vi "Autonomous.vi"   [LabVIEW 2015]
doc: "This VI starts when autonomous period begins, and will automatically be terminated when it ends. You can carry out timed or sensor driven operations directly to I/O or to subsystems without needing to return to the caller."
uses:
  <vilib>/Rock Robotics/WPI/CAN/TalonSRX/WPI_CANTalonSRX_Params.ctl
  <vilib>/Rock Robotics/Network Tables/NT Read Number.vi
  <vilib>/Rock Robotics/Network Tables/NT Read Boolean.vi
  Drive/Implementation/Drive Published Globals.vi
  Intake/Implementation/Intake Published Globals.vi
  Turret/Implementation/Turret Published Globals.vi
types:
  T1 = typedef "WPI_MotorControlDeviceRef.ctl" = cluster{"DeviceStatus":errorcluster, "Type":T2, "PWM":cluster{"PWM Channel":T3, "DeadBand":T4}, "CAN":cluster{"Device Number":u8, "Control Mode":T5, "Semaphore":T6, "Max Vout":dbl, "TalonSRX Control Mode":T7}, "Invert":bool}
  T2 = typedef "WPI_MotorControlType.ctl" = enum16{"PWM", "CAN", "CANTalonSRX"}
  T3 = typedef "FPGA_DIOPWMChannel.ctl" = enum8{"PWM 0", "PWM 1", "PWM 2", "PWM 3", "PWM 4", "PWM 5", "PWM 6", "PWM 7", "PWM 8", "PWM 9", "PWM MXP 0", "PWM MXP 1", "PWM MXP 2", "PWM MXP 3", "PWM MXP 4", "PWM MXP 5", "PWM MXP 6", "PWM MXP 7", "PWM MXP 8", "PWM MXP 9", "Invalid"}
  T4 = typedef "WPI_PWMDeadband.ctl" = cluster{"Name":string, "maxPositivePwm":i32, "minPositivePwm":i32, "centerPwm":i32, "maxNegativePwm":i32, "minNegativePwm":i32, "angularRange":u16}
  T5 = typedef "WPI_CANJaguar_ControlMode.ctl" = enum8{"Percent VBus", "Current", "Speed", "Position", "Voltage"}
  T6 = typedef "Semaphore RefNum" = refnum<k1>
  T7 = typedef "WPI_CANTalonSRX_APIControlMode.ctl" = enum8{"Percent VBus", "Speed", "Position", "Slave", "Unchanged / Invalid", "Voltage Compensation", "Current", "Motion Profile"}
  T8 = typedef "WPI_CANTalonSRX_Params.ctl" = u8
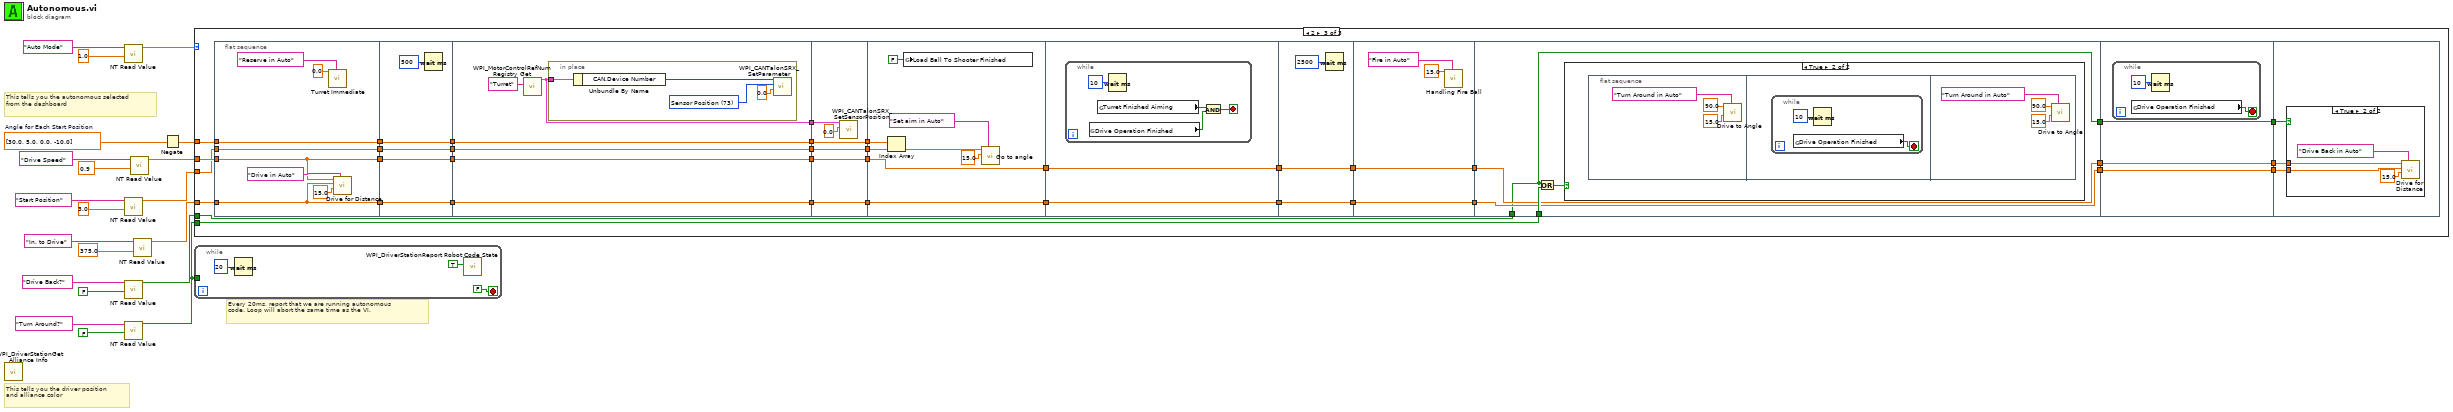
[diagram p0: block diagram]
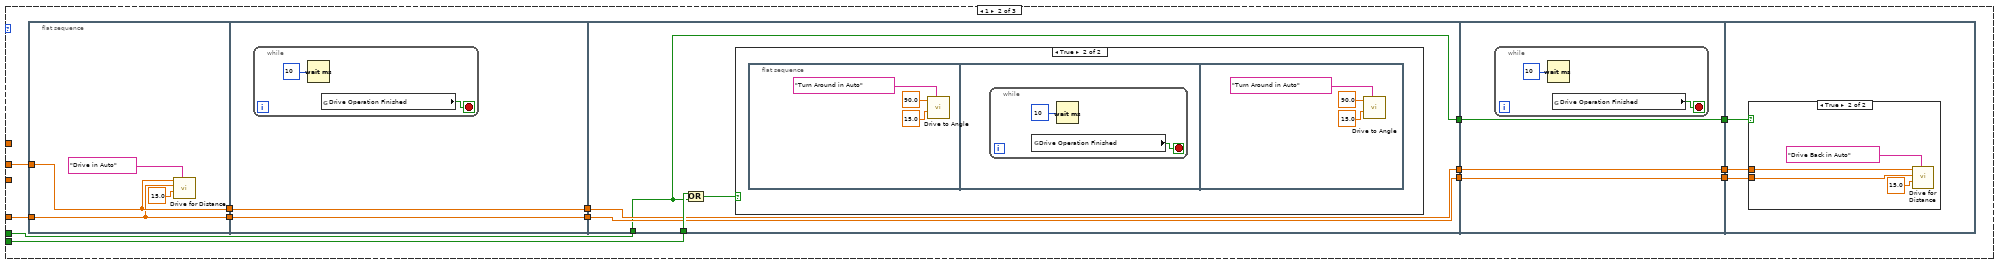
[diagram p3: hidden frame]
diagram:
  w13 = dbl[] [30.0, 5.0, 0.0, -10.0]  # Angle for Each Start Position
  # "This tells you the autonomous selected\nfrom the dashboard"
  # "Every 20ms, report that we are running autonomous\ncode. Loop will abort the same time as the VI."
  # "This tells you the driver position\nand alliance color"
  n1 = call <vilib>:"WPI_DriverStationGet Alliance Info.vi"() -> ()  [unwired: 12 out]
  n2 = call-poly <vilib>:"NT Read Value.vi"("Default Value"=1.0, "Name"="Auto Mode") -> ("Numeric"=w19:dbl)  [unwired: 8 in, 1 out]
  n3 = call-poly <vilib>:"NT Read Value.vi"("Default Value"=3.0, "Name"="Start Position") -> ("Numeric"=w12:dbl)  [unwired: 8 in, 1 out]
  n4 = call-poly <vilib>:"NT Read Value.vi"("Default Value"=FALSE, "Name"="Drive Back?") -> ("Boolean"=w3:bool)  [unwired: 8 in, 1 out]
  n5 = call-poly <vilib>:"NT Read Value.vi"("Default Value"=FALSE, "Name"="Turn Around?") -> ("Boolean"=w1:bool)  [unwired: 8 in, 1 out]
  n6 = call-poly <vilib>:"NT Read Value.vi"("Default Value"=0.9, "Name"="Drive Speed") -> ("Numeric"=w15:dbl)  [unwired: 8 in, 1 out]
  n7 = call-poly <vilib>:"NT Read Value.vi"("Default Value"=375.0, "Name"="In. to Drive") -> ("Numeric"=w17:dbl)  [unwired: 8 in, 1 out]
  n8 = Negate(x=w13) -> (-x=w2:dbl[])
  n9 = case shown="2" w19 {
    tunnel: w17 -> [_ w34 w103]
    tunnel: w15 -> [_ w33 w104]
    tunnel: w2 -> [_ _ w102]
    tunnel: w12 -> [_ _ w101]
    tunnel: w1 -> [_ w32 w99]
    tunnel: w3 -> [_ w31 w100]
    frame 0, Default {
    }
    frame 1 {
      n10 = flat-sequence {
        tunnel: w34 -> [w35]
        tunnel: w33 -> [w36]
        tunnel: [w36] -> w30
        tunnel: [w35] -> w28
        tunnel: w30 -> [w40]
        tunnel: [w40] -> w29
        tunnel: w28 -> [w39]
        tunnel: [w39] -> w27
        tunnel: w32 -> [w47]
        tunnel: w31 -> [w44]
        tunnel: w29 -> [w46]
        tunnel: [w46] -> w26
        tunnel: w27 -> [w45]
        tunnel: [w45] -> w24
        tunnel: [w44] -> w22
        tunnel: w26 -> [w58]
        tunnel: [w58] -> w25
        tunnel: w24 -> [w57]
        tunnel: [w57] -> w23
        tunnel: w22 -> [w56]
        tunnel: [w56] -> w21
        tunnel: w25 -> [w63]
        tunnel: w23 -> [w62]
        tunnel: w21 -> [w61]
        frame #0 {
          n11 = call "Drive for Distance.vi"("Description"="Drive in Auto", "Duration"=15.0, "Distance (in.)"=w35, "Speed (-1 to 1)"=w36) -> ()  [unwired: 7 in, 1 out]
        }
        frame #1 {
          n12 = while {
            stop <- w41 stop-if-true
            n13 = Wait (ms)(milliseconds to wait=10) -> ()  [unwired: 1 out]
            n14 = global read "Drive Published Globals.vi" "Drive Operation Finished"() -> (w41:bool)
          }
        }
        frame #2 {
          n15 = Or(x=w47, y=w44) -> (x .or. y?=w43:bool)
          n16 = case shown="True" w43 {
            frame False {
            }
            frame True {
              n17 = flat-sequence {
                frame #0 {
                  n18 = call "Drive to Angle.vi"("Description"="Turn Around in Auto", "Duration"=15.0, "Angle"=90.0) -> ()  [unwired: 8 in, 1 out]
                }
                frame #1 {
                  n19 = while {
                    stop <- w51 stop-if-true
                    n20 = global read "Drive Published Globals.vi" "Drive Operation Finished"() -> (w51:bool)
                    n21 = Wait (ms)(milliseconds to wait=10) -> ()  [unwired: 1 out]
                  }
                }
                frame #2 {
                  n22 = call "Drive to Angle.vi"("Description"="Turn Around in Auto", "Duration"=15.0, "Angle"=90.0) -> ()  [unwired: 8 in, 1 out]
                }
              }
            }
          }
        }
        frame #3 {
          n23 = while {
            stop <- w59 stop-if-true
            n24 = Wait (ms)(milliseconds to wait=10) -> ()  [unwired: 1 out]
            n25 = global read "Drive Published Globals.vi" "Drive Operation Finished"() -> (w59:bool)
          }
        }
        frame #4 {
          n26 = case shown="True" w61 {
            tunnel: w63 -> [_ w65]
            tunnel: w62 -> [_ w64]
            frame False {
            }
            frame True {
              n27 = call "Drive for Distance.vi"("Description"="Drive Back in Auto", "Duration"=15.0, "Distance (in.)"=w64, "Speed (-1 to 1)"=w65) -> ()  [unwired: 7 in, 1 out]
            }
          }
        }
      }
    }
    frame 2 {
      n28 = flat-sequence {
        tunnel: w101 -> [w111]
        tunnel: w102 -> [w112]
        tunnel: w103 -> [w108]
        tunnel: w104 -> [w107]
        tunnel: [w107] -> w84
        tunnel: [w108] -> w82
        tunnel: [w112] -> w80
        tunnel: [w111] -> w78
        tunnel: w84 -> [w117]
        tunnel: [w117] -> w83
        tunnel: w82 -> [w116]
        tunnel: [w116] -> w81
        tunnel: w80 -> [w115]
        tunnel: [w115] -> w79
        tunnel: w78 -> [w114]
        tunnel: [w114] -> w77
        tunnel: [w123] -> w76
        tunnel: [w122] -> w74
        tunnel: [w121] -> w72
        tunnel: [w120] -> w70
        tunnel: w83 -> [w123]
        tunnel: w81 -> [w122]
        tunnel: w79 -> [w121]
        tunnel: w77 -> [w120]
        tunnel: [w118] -> w68
        tunnel: w76 -> [w133]
        tunnel: [w133] -> w75
        tunnel: w74 -> [w132]
        tunnel: [w132] -> w73
        tunnel: w72 -> [w131]
        tunnel: [w131] -> w71
        tunnel: w70 -> [w130]
        tunnel: [w130] -> w69
        tunnel: w68 -> [w129]
        tunnel: w75 -> [w135]
        tunnel: w73 -> [w134]
        tunnel: w71 -> [w141]
        tunnel: w69 -> [w140]
        tunnel: [w135] -> w95
        tunnel: [w134] -> w91
        tunnel: [w143] -> w96
        tunnel: w95 -> [w143]
        tunnel: [w142] -> w92
        tunnel: w91 -> [w142]
        tunnel: [w149] -> w97
        tunnel: w96 -> [w149]
        tunnel: [w148] -> w93
        tunnel: w92 -> [w148]
        tunnel: [w152] -> w98
        tunnel: w97 -> [w152]
        tunnel: [w151] -> w94
        tunnel: w93 -> [w151]
        tunnel: w100 -> [w155]
        tunnel: w99 -> [w158]
        tunnel: w98 -> [w157]
        tunnel: w94 -> [w156]
        tunnel: [w155] -> w90
        tunnel: [w157] -> w89
        tunnel: [w156] -> w88
        tunnel: w90 -> [w170]
        tunnel: [w170] -> w87
        tunnel: w89 -> [w169]
        tunnel: [w169] -> w86
        tunnel: w88 -> [w168]
        tunnel: [w168] -> w85
        tunnel: w85 -> [w173]
        tunnel: w86 -> [w174]
        tunnel: w87 -> [w175]
        frame #0 {
          n29 = call "Turret Immediate.vi"("Description"="Reserve in Auto", "Speed (-1 to 1)"=0.0) -> ()  [unwired: 9 in, 1 out]
          n30 = call "Drive for Distance.vi"("Description"="Drive in Auto", "Duration"=15.0, "Distance (in.)"=w108, "Speed (-1 to 1)"=w107) -> ()  [unwired: 7 in, 1 out]
        }
        frame #1 {
          n31 = Wait (ms)(milliseconds to wait=500) -> ()  [unwired: 1 out]
        }
        frame #2 {
          n32 = call <vilib>:"WPI_MotorControlRefNum Registry Get.vi"("refnum name"="Turret") -> ("MotorControlDevRef"=w118:T1)  [unwired: 9 in, 1 out]
          n33 = in-place {
            in-place-border: w118 -> [w127]
            w125 = T8 73 items=["Slot 0 - P"=1, "Slot 0 - I"=2, "Slot 0 - D"=3, "Slot 0 - F"=4, "Slot 0 - I Zone"=5, "Slot 0 - Ramp Rate"=6, "Slot 1 - P"=11, "Slot 1 - I"=12, "Slot 1 - D"=13, "Slot 1 - F"=14, "Slot 1 - I Zone"=15, "Slot 1 - Ramp Rate"=16, "Soft Limit - Forward"=21, "Soft Limit - Reverse"=22, "On Boot - Brake Mode"=31, "On Boot - Limit Normally Closed - Forward"=32, "On Boot - Limit Normally Closed - Reverse"=33, "On Boot - Limit Disabled - Forward"=34, "On Boot - Limit Disabled - Reverse"=35, "Fault - Over Temp"=41, "Fault - Under Voltage"=42, "Fault - Forward Limit"=43, "Fault - Reverse Limit"=44, "Fault - Hardware Failure"=45, "Fault - Forward Soft Limit"=46, "Fault - Reverse Soft Limit"=47, "Sticky Fault - Over Temp"=48, "Sticky Fault - Under Voltage"=49, "Sticky Fault - Forward Limit"=50, "Sticky Fault - Reverse Limit"=51, "Sticky Fault - Forward Soft Limit"=52, "Sticky Fault - Reverse Soft Limit"=53, "Applied Throttle"=61, "Closed-Loop Error"=62, "Select Feedback Device"=63, "Reverse Closed-Loop Output"=64, "Mode Select"=65, "Profile Slot Select"=66, "Ramp Throttle"=67, "Reverse Feedback Sensor"=68, "Limit Switch Enabled"=69, "Limit Switch Closed - Forward"=70, "Limit Switch Closed - Reverse"=71, "Sensor Position"=73, "Sensor Velocity"=74, "Current"=75, "Brake is Enabled"=76, "Encoder Position"=77, "Encoder Velocity"=78, "Encoder Index Rise Events"=79, "Encoder A Pin State"=80, "Encoder B Pin State"=81, "Encoder Index Pin State"=82, "Analog In with Overflow"=83, "Analog In Velocity"=84, "Temperature"=85, "Battery Voltage"=86, "Reset Count"=87, "Reset Flags"=88, "Firmware Version"=89, "Settings Changed"=90] ("Parameter")
            n34 = Unbundle By Name(w127) -> ("CAN.Device Number"=w126:u8)
            n35 = call <vilib>:"WPI_CANTalonSRX_SetParameter.vi"("Value"=0.0, "Parameter"=w125, "Device ID (0)"=w126) -> ()  [unwired: 7 in, 2 out]
          }
        }
        frame #3 {
          n36 = call <vilib>:"WPI_CANTalonSRX_SetSensorPosition.vi"("New Sensor Position"=0.0, "CAN Talon SRX Ref"=w129) -> ()  [unwired: 8 in, 2 out]
        }
        frame #4 {
          n37 = Index Array(array=w141, index=w140) -> (element=w139:dbl)
          n38 = global write "Intake Published Globals.vi" "Load Ball To Shooter Finished"(FALSE) -> ()
          n39 = call "Go to angle.vi"("Description"="Set aim in Auto", "Duration"=15.0, "Angle  (degrees, 0=straight ahead)"=w139) -> ()  [unwired: 8 in, 1 out]
        }
        frame #5 {
          n40 = while {
            stop <- w145 stop-if-true
            n41 = global read "Drive Published Globals.vi" "Drive Operation Finished"() -> (w147:bool)
            n42 = global read "Turret Published Globals.vi" "Turret Finished Aiming"() -> (w146:bool)
            n43 = Wait (ms)(milliseconds to wait=10) -> ()  [unwired: 1 out]
            n44 = And(x=w146, y=w147) -> (x .and. y?=w145:bool)
          }
        }
        frame #6 {
          n45 = Wait (ms)(milliseconds to wait=2500) -> ()  [unwired: 1 out]
        }
        frame #7 {
          n46 = call "Handling Fire Ball.vi"("Description"="Fire in Auto", "Duration"=15.0) -> ()  [unwired: 9 in, 1 out]
        }
        frame #8 {
          n47 = Or(x=w155, y=w158) -> (x .or. y?=w159:bool)
          n48 = case shown="True" w159 {
            frame False {
            }
            frame True {
              n49 = flat-sequence {
                frame #0 {
                  n50 = call "Drive to Angle.vi"("Description"="Turn Around in Auto", "Duration"=15.0, "Angle"=90.0) -> ()  [unwired: 8 in, 1 out]
                }
                frame #1 {
                  n51 = while {
                    stop <- w163 stop-if-true
                    n52 = global read "Drive Published Globals.vi" "Drive Operation Finished"() -> (w163:bool)
                    n53 = Wait (ms)(milliseconds to wait=10) -> ()  [unwired: 1 out]
                  }
                }
                frame #2 {
                  n54 = call "Drive to Angle.vi"("Description"="Turn Around in Auto", "Duration"=15.0, "Angle"=90.0) -> ()  [unwired: 8 in, 1 out]
                }
              }
            }
          }
        }
        frame #9 {
          n55 = while {
            stop <- w171 stop-if-true
            n56 = global read "Drive Published Globals.vi" "Drive Operation Finished"() -> (w171:bool)
            n57 = Wait (ms)(milliseconds to wait=10) -> ()  [unwired: 1 out]
          }
        }
        frame #10 {
          n58 = case shown="True" w175 {
            tunnel: w174 -> [_ w179]
            tunnel: w173 -> [_ w178]
            frame False {
            }
            frame True {
              n59 = call "Drive for Distance.vi"("Description"="Drive Back in Auto", "Duration"=15.0, "Distance (in.)"=w178, "Speed (-1 to 1)"=w179) -> ()  [unwired: 7 in, 1 out]
            }
          }
        }
      }
    }
  }
  n60 = while {
    tunnel: w1 -> [_]
    stop <- FALSE stop-if-true
    n61 = Wait (ms)(milliseconds to wait=u32 20) -> ()  [unwired: 1 out]
    n62 = call <vilib>:"WPI_DriverStationReport Robot Code State.vi"("Autonomous"=TRUE) -> ()  [unwired: 10 in, 1 out]
  }
